vi "binning.vi"(1 "y binning":u8, 2 "x binning":u8, 3 "Average?":bool, 4 "data in":dbl[][](array[numeric])) -> (0 "data out":dbl[][](array[numeric]))   [LabVIEW 2015]
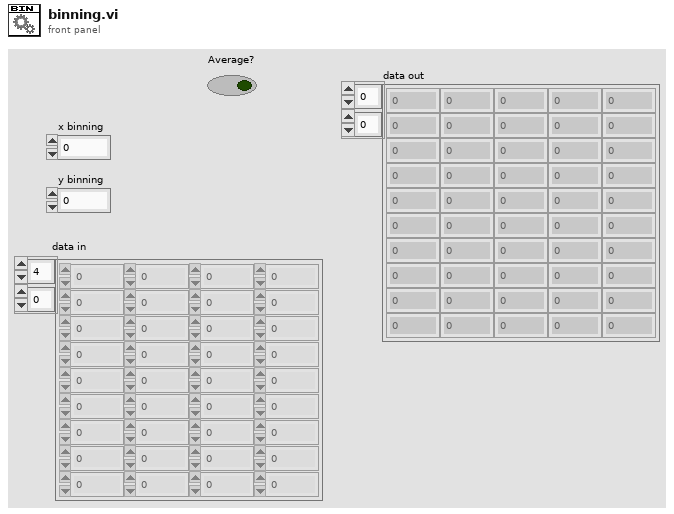
[diagram p1: front panel]
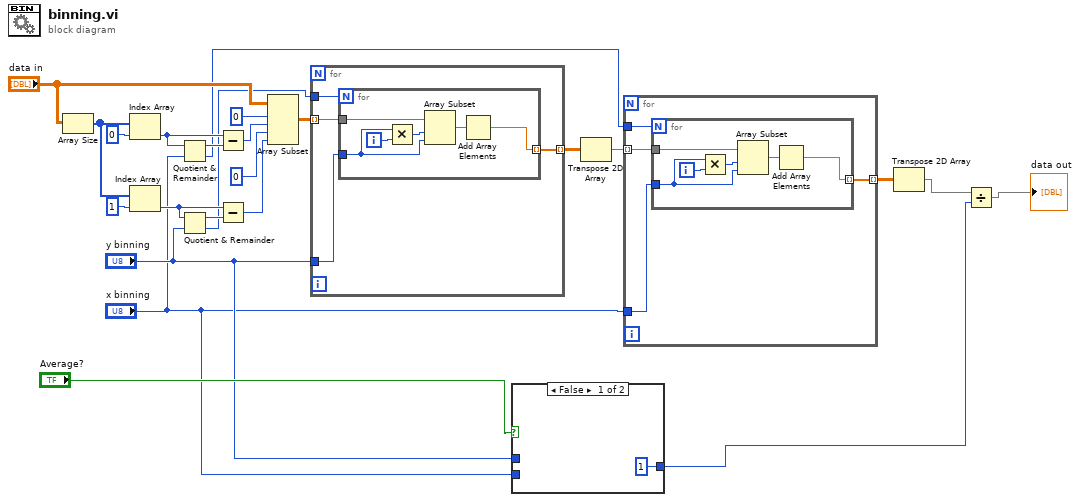
[diagram p0: block diagram]
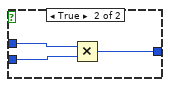
[diagram p2: hidden frame]
diagram:
  n1 = Array Size(array="data in") -> (size(s)=w22:i32[])
  n2 = Index Array(array=w22, index=0 ("索引")) -> (element=w18:i32)
  n3 = Index Array(array=w22, index=1 ("索引")) -> (element=w16:i32)
  n4 = Quotient & Remainder(x=w18, y="x binning") -> (x-y*floor(x/y)=w17:i32, floor(x/y)=w7:i32)
  n5 = Quotient & Remainder(x=w16, y="y binning") -> (x-y*floor(x/y)=w15:i32, floor(x/y)=w8:i32)
  n6 = Subtract(x=w18, y=w17) -> (x-y=w14:i32)
  n7 = Subtract(x=w16, y=w15) -> (x-y=w13:i32)
  n8 = Array Subset(array="data in", index (row)=0 ("索引"), length (row)=w14, index (col)=0 ("索引"), length (col)=w13) -> (w12:dbl[][])
  n9 = for {
    tunnel: w12 -> [w27] mode=indexing
    tunnel: w8 -> [w28]
    tunnel: "y binning" -> [w26]
    tunnel: [w25] -> w11 mode=indexing
    n10 = for {
      N: w28 -> [_]
      tunnel: w27 -> [w32]
      tunnel: w26 -> [w30]
      tunnel: [w29] -> w25 mode=indexing
      i -> [w34]
      n11 = Multiply(x=w30, y=w34) -> (x*y=w33:i32)
      n12 = Array Subset(array=w32, index=w33, length=w30) -> (w31:dbl[])
      n13 = Add Array Elements(numeric array=w31) -> (sum=w29:dbl)
    }
  }
  n14 = case shown="False" "Average?" {
    tunnel: "y binning" -> [_ w38]
    tunnel: "x binning" -> [_ w37]
    tunnel: [u8 1 w36] -> w1
    frame False {
    }
    frame True {
      n15 = Multiply(x=w38, y=w37) -> (x*y=w36:u8)
    }
  }
  n16 = Transpose 2D Array(2D array=w11) -> (transposed array=w10:dbl[][])
  n17 = for {
    tunnel: w7 -> [w42]
    tunnel: "x binning" -> [w41]
    tunnel: [w40] -> w9 mode=indexing
    tunnel: w10 -> [w39] mode=indexing
    n18 = for {
      N: w42 -> [_]
      tunnel: w39 -> [w46]
      tunnel: w41 -> [w44]
      tunnel: [w43] -> w40 mode=indexing
      i -> [w48]
      n19 = Multiply(x=w44, y=w48) -> (x*y=w47:i32)
      n20 = Array Subset(array=w46, index=w47, length=w44) -> (w45:dbl[])
      n21 = Add Array Elements(numeric array=w45) -> (sum=w43:dbl)
    }
  }
  n22 = Transpose 2D Array(2D array=w9) -> (transposed array=w6:dbl[][])
  n23 = Divide(x=w6, y=w1) -> (x/y=→"data out":dbl[][])
